vi "vi server center window.vi"(0 "VI ref in":refnum<vi>, 11 "error in":errorcluster) -> (4 "VI ref out":refnum<vi>, 8 "Front Panel Window:Window Bounds":T1, 15 "error out":errorcluster)   [LabVIEW 2016]
doc: "This vi centers the window for a given vi reference.\n\nPaul K Dixon\nPhysics 350\nCSUSB Physics"
uses:
  <vilib>/Utility/miscctls.llb/LVRectTypeDef.ctl
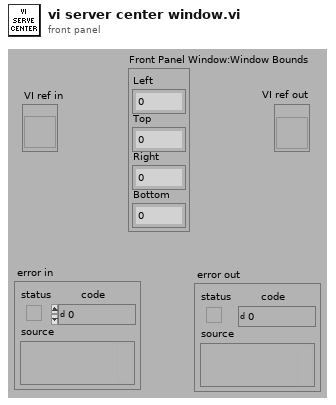
[diagram p1: front panel]
types:
  T1 = typedef "LVRectTypeDef.ctl" = cluster{"Left":i16, "Top":i16, "Right":i16, "Bottom":i16}
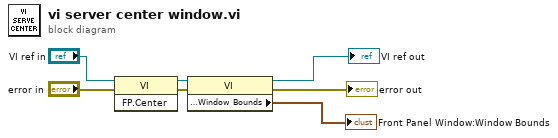
[diagram p0: block diagram]
diagram:
  n1 = invoke class="VI" method="FP.Center"(reference="VI ref in", error in="error in") -> (reference out=w4:refnum<vi>, error out=w5:errorcluster)  [unwired: 1 in, 1 out]
  n2 = property class="VI"(reference=w4, error in=w5) -> (reference out=→"VI ref out":refnum<vi>, error out=→"error out":errorcluster, "Front Panel Window:Window Bounds"=→"Front Panel Window:Window Bounds":T1)
